vi "csm_lumikki_instron_creep.vi"(8 "creepLoad":dbl, 9 "channelInt":i32) -> (0 "creepLoadOut":dbl, 1 "channelIntOut":i32, 2 "creepRunningOut":bool, 3 "startCreepOut":bool)   [LabVIEW 2009]
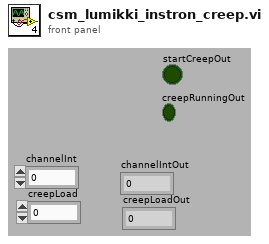
[diagram p1: front panel]
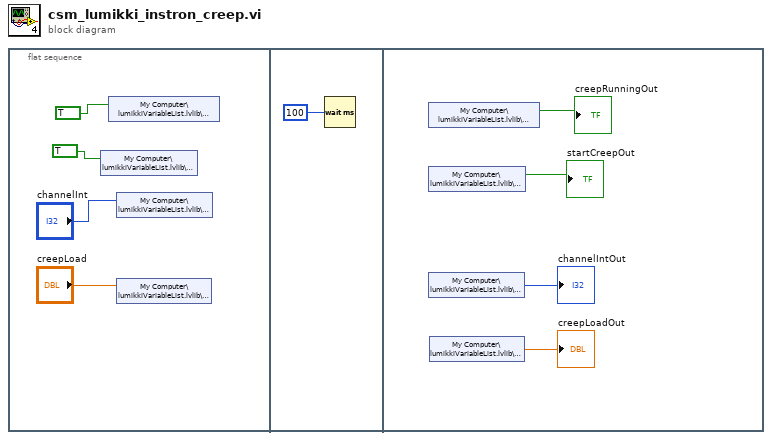
[diagram p0: block diagram]
diagram:
  n1 = flat-sequence {
    frame #0 {
      n2 = shared-variable "My Computer\\lumikkiVariableList.lvlib\\startCreep"(TRUE ("Busy")) -> ()  [unwired: 1 in, 1 out]
      n3 = shared-variable "My Computer\\lumikkiVariableList.lvlib\\creepRunning"(TRUE ("Busy")) -> ()  [unwired: 1 in, 1 out]
      n4 = shared-variable "My Computer\\lumikkiVariableList.lvlib\\channelInt"("channelInt") -> ()  [unwired: 1 in, 1 out]
      n5 = shared-variable "My Computer\\lumikkiVariableList.lvlib\\creepLoad"("creepLoad") -> ()  [unwired: 1 in, 1 out]
    }
    frame #1 {
      n6 = Wait (ms)(milliseconds to wait=u32 100) -> ()  [unwired: 1 out]
    }
    frame #2 {
      n7 = shared-variable "My Computer\\lumikkiVariableList.lvlib\\creepRunning"() -> (→"creepRunningOut":bool)  [unwired: 1 in, 1 out]
      n8 = shared-variable "My Computer\\lumikkiVariableList.lvlib\\startCreep"() -> (→"startCreepOut":bool)  [unwired: 1 in, 1 out]
      n9 = shared-variable "My Computer\\lumikkiVariableList.lvlib\\channelInt"() -> (→"channelIntOut":i32)  [unwired: 1 in, 1 out]
      n10 = shared-variable "My Computer\\lumikkiVariableList.lvlib\\creepLoad"() -> (→"creepLoadOut":dbl)  [unwired: 1 in, 1 out]
    }
  }
